vi "Manage Drive.vi"(7 "Min Drive Free Space (%)":dbl, 8 "error in":errorcluster, 11 "Data Folder":path=path "c:/data") -> (0 "error out":errorcluster, 2 "Drive Space Below Limit":bool)   [LabVIEW 2022 SP3]
uses:
  Globals/Global - Monitoring Variables.vi
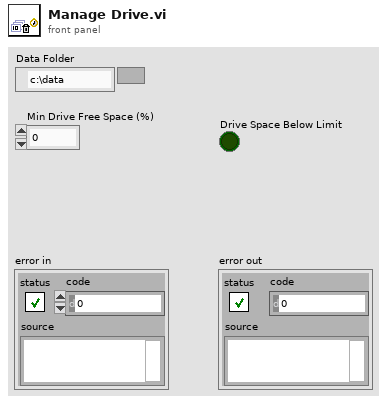
[diagram p1: front panel]
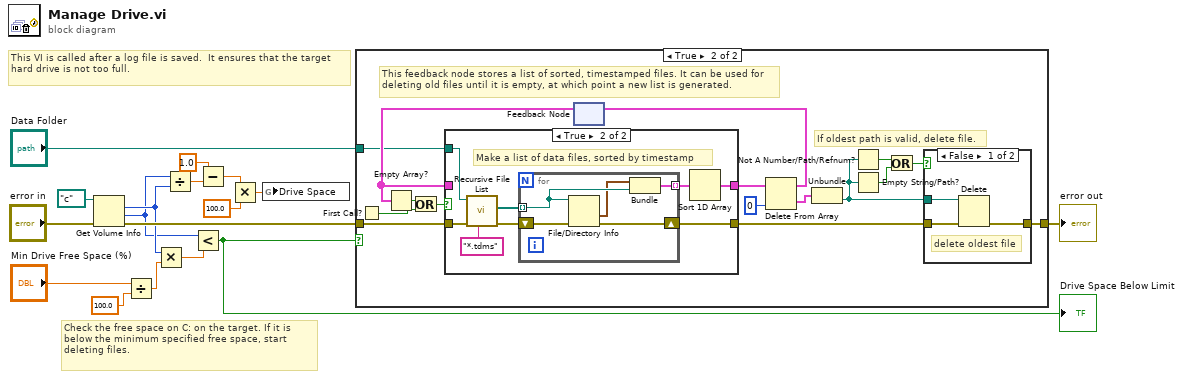
[diagram p0: block diagram]
diagram:
  # "Check the free space on C: on the target. If it is below the minimum specified free space, start deleting files."
  # "This VI is called after a log file is saved.  It ensures that the target hard drive is not too full."
  n1 = Get Volume Info(8:"error in", 11:path "c:/" ("path")) -> (0:w10:errorcluster, 1:w7:i64, 2:w8:i64)  [unwired: 3 out]
  n2 = Divide(x="Min Drive Free Space (%)", y=100.0) -> (x/y=w14:dbl)
  n3 = Multiply(x=w8, y=w14) -> (x*y=w17:dbl)
  n4 = Divide(x=w7, y=w8) -> (x/y=w6:dbl)
  n5 = Less?(x=w7, y=w17) -> (x < y?=w11:bool)
  "Drive Space Below Limit" <- w11
  n6 = Subtract(x=1.0, y=w6) -> (x-y=w3:dbl)
  n7 = Multiply(x=w3, y=100.0) -> (x*y=w4:dbl)
  n8 = global write "Global - Monitoring Variables.vi" "Drive Space"(w4) -> ()
  n9 = case shown="True" w11 {
    tunnel: w10 -> [w18 w34]
    tunnel: [w18 w29] -> w9
    tunnel: "Data Folder" -> [_ w25]
    frame False {
      # "Free space is not below the minimum threshold.  Do nothing."
    }
    frame True {
      # "If oldest path is valid, delete file."
      # "This feedback node stores a list of sorted, timestamped files. It can be used for deleting old files until it is empty, at which point a new list is generated."
      n10 = First Call?() -> (First Call?: T/F=w32:bool)
      n11 = feedback #1() -> (w27:cluster{"last mod":timestamp, path}[])  [unwired: 1 out]
      n12 = Empty Array?(array=w27) -> (empty?=w26:bool)
      n13 = Or(x=w26, y=w32) -> (x .or. y?=w33:bool)
      n14 = case shown="True" w33 {
        tunnel: w34 -> [w40 w48]
        tunnel: [w40 w44] -> w28
        tunnel: [w39 w42] -> w31
        tunnel: w27 -> [w39 _]
        tunnel: w25 -> [_ w41]
        frame False {
          # "Current list of old files is non-empty.  Use it."
        }
        frame True {
          # "Make a list of data files, sorted by timestamp"
          n15 = call <vilib>:"Recursive File List.vi"("pattern"="*.tdms", "error in (no error)"=w48, "Folder Path"=w41) -> ("error out"=w45:errorcluster, "All Files in Dir"=w46:path[])  [unwired: 1 in, 6 out]
          n16 = for {
            tunnel: w46 -> [w50] mode=indexing
            shift-right: [w52] -> w44
            shift-left: w45 -> [w53]
            tunnel: [w51] -> w43 mode=indexing
            n17 = File/Directory Info(path=w50, error in=w53) -> (last mod=w49:timestamp, error out=w52:errorcluster)  [unwired: 5 out]
            n18 = Bundle("last mod"=w49, w50) -> (w51:cluster{"last mod":timestamp, path})  [unwired: 1 out]
          }
          n19 = Sort 1D Array(array=w43) -> (sorted array=w42:cluster{"last mod":timestamp, path}[])
        }
      }
      n20 = Delete From Array(array=w31, index=0) -> (deleted portion=w23:cluster{"last mod":timestamp, path}, array with subset deleted=w30:cluster{"last mod":timestamp, path}[])  [unwired: 1 in]
      n21 = feedback-in #1(w30) -> ()
      n22 = Unbundle(w23) -> (w22:path)  [unwired: 1 out]
      n23 = Not A Number/Path/Refnum?(number/path/refnum=w22) -> (NaN/Path/Refnum?=w21:bool)
      n24 = Empty String/Path?(string/path=w22) -> (empty?=w20:bool)
      n25 = Or(x=w21, y=w20) -> (x .or. y?=w19:bool)
      n26 = case shown="False" w19 {
        tunnel: [w37 w38] -> w29
        tunnel: w28 -> [w36 w38]
        tunnel: w22 -> [w35 _]
        frame False {
          # "delete oldest file"
          n27 = Delete(path (use dialog)=w35, error in=w36) -> (error out=w37:errorcluster)  [unwired: 5 out]
        }
        frame True {
        }
      }
    }
  }
  "error out" <- w9
